vi "String - Remove Quotation Marks From String.vi"(5 "String":string) -> (2 "result string":string)   [LabVIEW 2020]
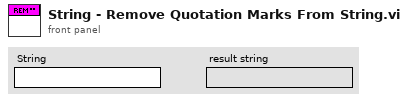
[diagram p1: front panel]
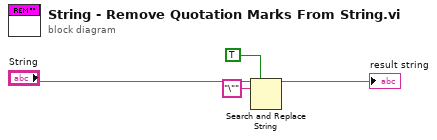
[diagram p0: block diagram]
diagram:
  n1 = Search and Replace String(replace all?=TRUE ("replace all? (F)"), input string="String", search string="\"") -> (result string=→"result string":string)  [unwired: 5 in, 3 out]
